vi "Close.vi"(8 "error in (no error)":errorcluster, 11 "VISA resource name":refnum<visa-resource-name>) -> (0 "error out":errorcluster)   [LabVIEW 2016, in "Andeen-Hagerling 2550.lvlib"]
doc: "Performs an instrument error query before terminating the software connection to the instrument."
uses:
  Andeen-Hagerling 2550.lvlib
  <vilib>/Instr/_visa.llb/VISA GPIB Control REN Mode.ctl
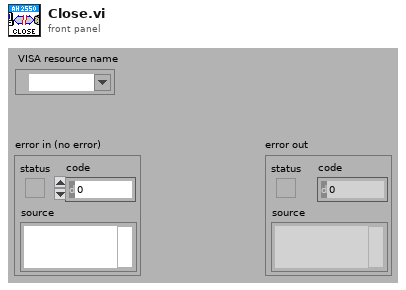
[diagram p1: front panel]
types:
  T1 = typedef "VISA GPIB Control REN Mode.ctl" = u16
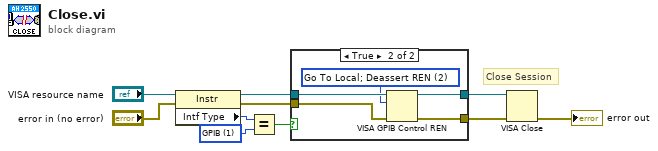
[diagram p0: block diagram]
diagram:
  w6 = u16 1 items=["GPIB"=1, "VXI"=2, "GPIB-VXI"=3, "Serial"=4, "PXI"=5, "TCPIP"=6, "USB"=7, "FireWire"=9] ("Interface Information:Interface Type")
  # "Close Session"
  n1 = property class="Instr"(reference="VISA resource name", error in="error in (no error)") -> (reference out=w5:refnum<visa-resource-name>, error out=w3:errorcluster, "Intf Type"=w7:u16)
  n2 = Equal?(x=w7, y=w6) -> (x = y?=w1:bool)
  n3 = case shown="True" w1 {
    tunnel: w5 -> [w12 w17]
    tunnel: [w12 w16] -> w4
    tunnel: w3 -> [w11 w15]
    tunnel: [w11 w14] -> w2
    frame False {
    }
    frame True {
      w13 = T1 2 items=["Deassert REN", "Assert REN", "Go To Local; Deassert REN ", "Assert REN; Address Device", "Local Lockout (Addressed Devices)", "Local Lockout (This Device)", "Go To Local"] ("Mode")
      n4 = VISA GPIB Control REN(8:w15, 10:w13, 11:w17) -> (0:w14:errorcluster, 3:w16:refnum<visa-resource-name>)
    }
  }
  n5 = VISA Close(VISA resource name=w4, error in (no error)=w2) -> (error out=→"error out":errorcluster)
